vi "areaTop.vi"(2 "Array":dbl[][](array[numeric])) -> (6 "1":dbl[][](array[numeric]), 7 "2":dbl[][](array[numeric]), 9 "3":dbl[][](array[numeric]), 10 "4":dbl[][](array[numeric]))   [LabVIEW 2011]
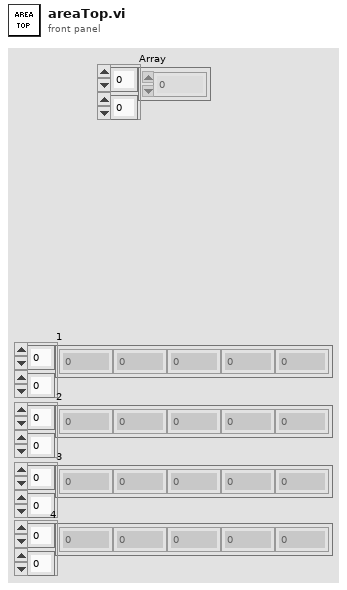
[diagram p1: front panel]
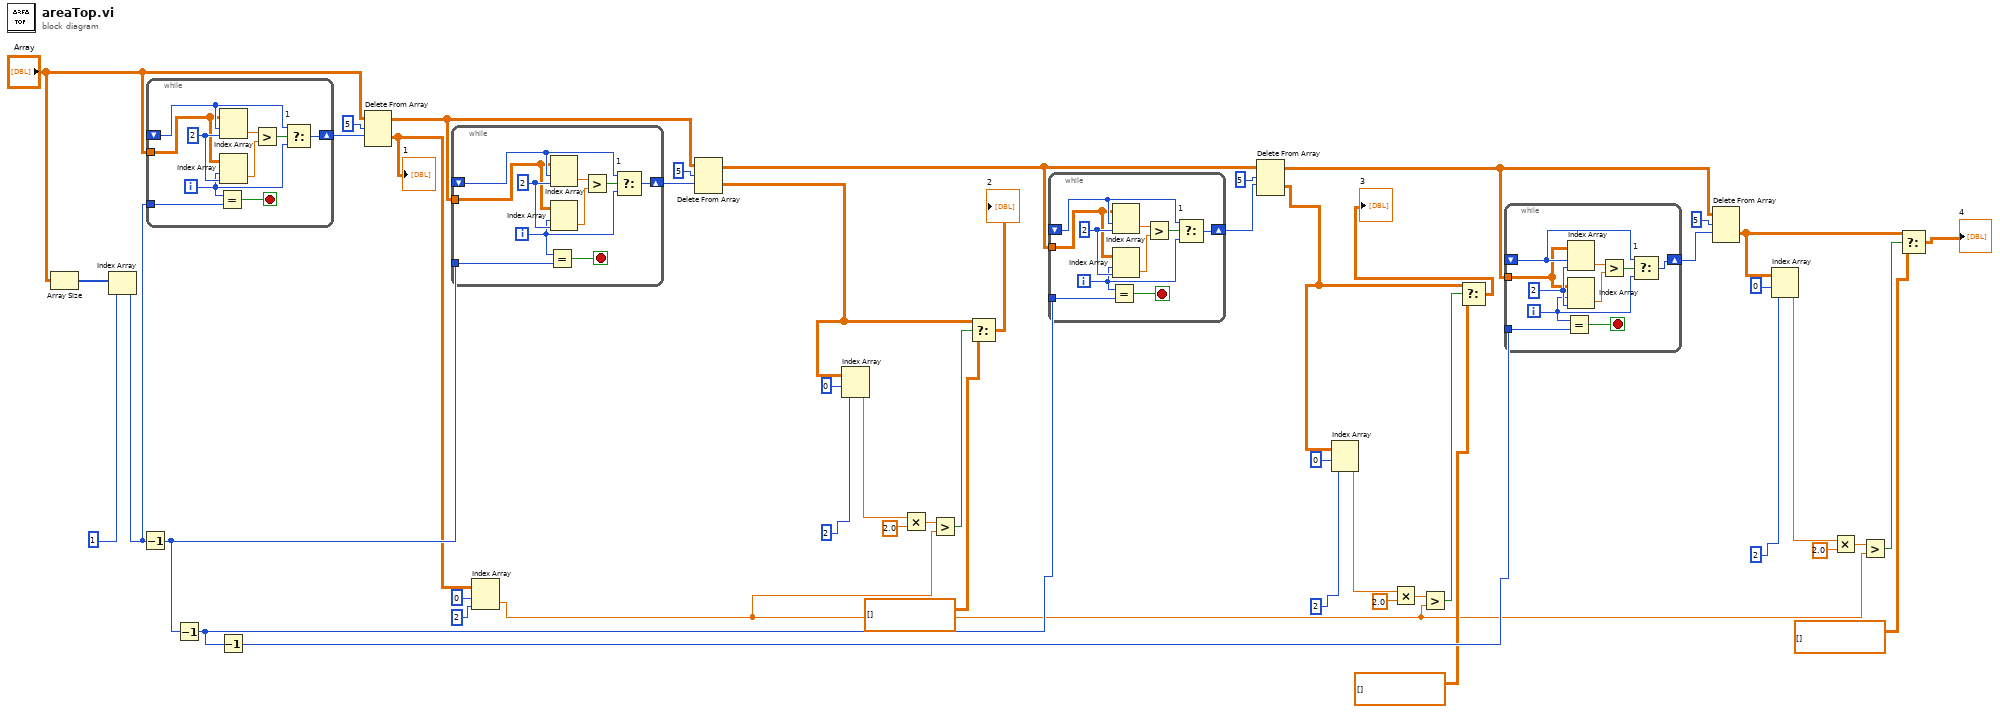
[diagram p0: block diagram]
diagram:
  n1 = Array Size(array="Array") -> (size(s)=w48:i32[])
  n2 = Index Array(array=w48, index=1) -> (element=w43:i32)
  n3 = Decrement(x=w43) -> (x-1=w38:i32)
  n4 = while {
    tunnel: w43 -> [w56]
    tunnel: "Array" -> [w52]
    shift-right: [w55] -> w46
    shift-left: _ -> [w58]
    i -> [w50]
    stop <- w59 stop-if-true
    w53 = 2 ("index (col)")
    n5 = Equal?(x=w50, y=w56) -> (x = y?=w59:bool)
    n6 = Index Array(array=w52, index (row)=w58, index (col)=w53) -> (element=w57:dbl)
    n7 = Index Array(array=w52, index (row)=w50, index (col)=w53) -> (element=w51:dbl)
    n8 = Greater?(x=w57, y=w51) -> (0:w54:bool)
    n9 = Select "1"(t=w58, s=w54, f=w50) -> (s? t:f=w55:i32)
  }
  n10 = Decrement(x=w38) -> (x-1=w33:i32)
  n11 = Decrement(x=w33) -> (x-1=w35:i32)
  n12 = Delete From Array(array="Array", length=5, index (row)=w46) -> (deleted portion=w25:dbl[][], array with subset deleted=w42:dbl[][])  [unwired: 1 in]
  "1" <- w25
  n13 = while {
    tunnel: w38 -> [w66]
    tunnel: w42 -> [w62]
    shift-right: [w65] -> w45
    shift-left: _ -> [w68]
    i -> [w60]
    stop <- w69 stop-if-true
    w63 = 2 ("index (col)")
    n14 = Equal?(x=w60, y=w66) -> (x = y?=w69:bool)
    n15 = Index Array(array=w62, index (row)=w68, index (col)=w63) -> (element=w67:dbl)
    n16 = Index Array(array=w62, index (row)=w60, index (col)=w63) -> (element=w61:dbl)
    n17 = Greater?(x=w67, y=w61) -> (0:w64:bool)
    n18 = Select "1"(t=w68, s=w64, f=w60) -> (s? t:f=w65:i32)
  }
  n19 = Index Array(array=w25, index (row)=0, index (col)=2 ("disabled index (col)")) -> (element=w2:dbl)
  n20 = Delete From Array(array=w42, length=5, index (row)=w45) -> (deleted portion=w4:dbl[][], array with subset deleted=w39:dbl[][])  [unwired: 1 in]
  n21 = Index Array(array=w4, index (row)=0, index (col)=2 ("disabled index (col)")) -> (element=w10:dbl)
  n22 = Multiply(x=w10, y=2.0) -> (x*y=w7:dbl)
  n23 = Greater?(x=w7, y=w2) -> (0:w5:bool)
  n24 = Select(t=w4, s=w5, f=dbl[][] []) -> (s? t:f=→"2":dbl[][])
  n25 = while {
    tunnel: w33 -> [w76]
    tunnel: w39 -> [w72]
    shift-right: [w75] -> w40
    shift-left: _ -> [w78]
    i -> [w70]
    stop <- w79 stop-if-true
    w73 = 2 ("index (col)")
    n26 = Equal?(x=w70, y=w76) -> (x = y?=w79:bool)
    n27 = Index Array(array=w72, index (row)=w78, index (col)=w73) -> (element=w77:dbl)
    n28 = Index Array(array=w72, index (row)=w70, index (col)=w73) -> (element=w71:dbl)
    n29 = Greater?(x=w77, y=w71) -> (0:w74:bool)
    n30 = Select "1"(t=w78, s=w74, f=w70) -> (s? t:f=w75:i32)
  }
  n31 = Delete From Array(array=w39, length=5, index (row)=w40) -> (deleted portion=w13:dbl[][], array with subset deleted=w34:dbl[][])  [unwired: 1 in]
  n32 = Index Array(array=w13, index (row)=0, index (col)=2 ("disabled index (col)")) -> (element=w19:dbl)
  n33 = Multiply(x=w19, y=2.0) -> (x*y=w16:dbl)
  n34 = Greater?(x=w16, y=w2) -> (0:w14:bool)
  n35 = Select(t=w13, s=w14, f=dbl[][] []) -> (s? t:f=→"3":dbl[][])
  n36 = while {
    tunnel: w35 -> [w86]
    tunnel: w34 -> [w82]
    shift-right: [w85] -> w37
    shift-left: _ -> [w88]
    i -> [w80]
    stop <- w89 stop-if-true
    w83 = 2 ("index (col)")
    n37 = Equal?(x=w80, y=w86) -> (x = y?=w89:bool)
    n38 = Index Array(array=w82, index (row)=w88, index (col)=w83) -> (element=w87:dbl)
    n39 = Index Array(array=w82, index (row)=w80, index (col)=w83) -> (element=w81:dbl)
    n40 = Greater?(x=w87, y=w81) -> (0:w84:bool)
    n41 = Select "1"(t=w88, s=w84, f=w80) -> (s? t:f=w85:i32)
  }
  n42 = Delete From Array(array=w34, length=5, index (row)=w37) -> (deleted portion=w21:dbl[][])  [unwired: 1 in, 1 out]
  n43 = Index Array(array=w21, index (row)=0, index (col)=2 ("disabled index (col)")) -> (element=w26:dbl)
  n44 = Multiply(x=w26, y=2.0) -> (x*y=w29:dbl)
  n45 = Greater?(x=w29, y=w2) -> (0:w31:bool)
  n46 = Select(t=w21, s=w31, f=dbl[][] []) -> (s? t:f=→"4":dbl[][])
